vi "Parse Text.vi"(8 "Error In":errorcluster) -> (0 "Error Out":errorcluster)   [LabVIEW 2018, in "Tests.lvlib" / "Parser.lvlib"]
uses:
  Parser.lvlib
  src/Toolkit/Tokens/Text/Text.lvclass
  src/Toolkit/Readers/String/String.lvclass
  D:/Users/cfield/Code/Field R&D Services/Mustache/trunk/src/Toolkit/Readers/Abstract/Abstract.lvclass
  <vilib>/Utility/LVClass/Get LV Class Name.vi
  src/Toolkit/Tokens/Text/API/Read Content.vi
  <vilib>/addons/_JKI Toolkits/Caraya/classes/Assert/Assert Equal_Variant.vi
  <vilib>/addons/_JKI Toolkits/Caraya/classes/Test/Test.lvclass
  src/Toolkit/Parser/Parser.lvclass
  <vilib>/addons/_JKI Toolkits/Caraya/classes/Assert/Assert.lvclass
  Tests.lvlib
  src/Toolkit/Tokens/Abstract/Abstract.lvclass
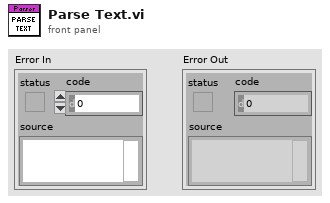
[diagram p1: front panel]
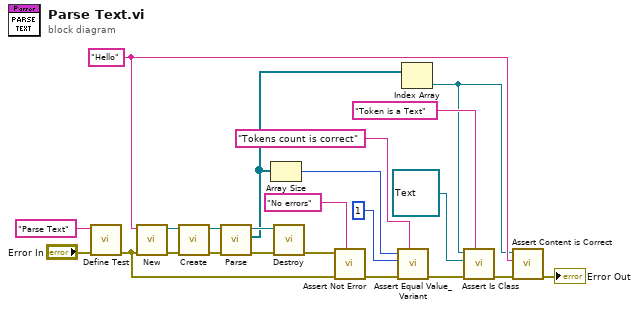
[diagram p0: block diagram]
diagram:
  w3 = "Hello" ("String")
  n1 = call <vilib>:"Define Test.vi"("error in (no error)"="Error In", "Label (VI Title)"="Parse Text") -> ("error out"=w14:errorcluster)  [unwired: 9 in]
  n2 = call "New.vi"("Error In"=w14, "String"=w3) -> ("Error Out"=w20:errorcluster, "String"=w21:refnum<class "String.lvclass">)  [unwired: 8 in]
  n3 = call "Create.vi"("Error In"=w20, "Reader"=w21) -> ("Error Out"=w19:errorcluster, "Parser"=w18:refnum<class "Parser.lvclass">)  [unwired: 8 in]
  n4 = call "Parse.vi"("Error In"=w19, "Parser In"=w18) -> ("Error Out"=w16:errorcluster, "Tokens"=w8:refnum<class "Abstract.lvclass">[], "Parser Out"=w17:refnum<class "Parser.lvclass">)  [unwired: 7 in]
  n5 = Array Size(array=w8) -> (size(s)=w10:i32)
  n6 = call "Destroy.vi"("Error In"=w16, "Parser"=w17) -> ("Error Out"=w15:errorcluster)  [unwired: 8 in, 1 out]
  n7 = call <vilib>:"Assert Not Error.vi"("Label"="No errors", "error in (no error)"=w14, "Not Error?"=w15) -> ("error out"=w12:errorcluster)  [unwired: 8 in]
  n8 = call <vilib>:"Assert Equal Value_Variant.vi"("Label"="Tokens count is correct", "error in (no error)"=w12, "Y"=1 ("size(s)"), "X"=w10) -> ("error out"=w7:errorcluster)  [unwired: 7 in]
  n9 = Index Array(array=w8) -> (element=w1:refnum<class "Abstract.lvclass">)  [unwired: 1 in]
  n10 = call "Assert Is Class.vi"("Label"="Token is a Text", "Error In"=w7, "Expected"=refnum<class "Text.lvclass"> refnum ("Mustache.lvlib:Tokens.lvlib:Text.lvclass"), "Actual"=w1) -> ("Error Out"=w2:errorcluster)  [unwired: 7 in]
  n11 = call "Assert Content is Correct.vi"("Error In"=w2, "Expected"=w3, "Token"=w1) -> ("Error Out"=→"Error Out":errorcluster)  [unwired: 8 in]
